vi "1WIRE_pulll_up_for_convert.vi"(8 "error in":errorcluster) -> (0 "error out":errorcluster)   [LabVIEW 2013]
doc: "This VI is created by Vincent Claes for FPDA-1 more information on http://pwo.fpga.be\n\nvincent.claes@xios.be\nclaesvincent@gmail.com\n\nhttp://www.linkedin.com/in/vincentclaes"
uses:
  <vilib>/eio/EIONode/EIONode.xnode
  <vilib>/eio/EIOMethodNode/EIOMethodNode.xnode
  <vilib>/rvi/eio/common/nirviEmuTemplateMethod_errors.vi
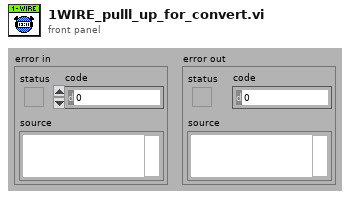
[diagram p1: front panel]
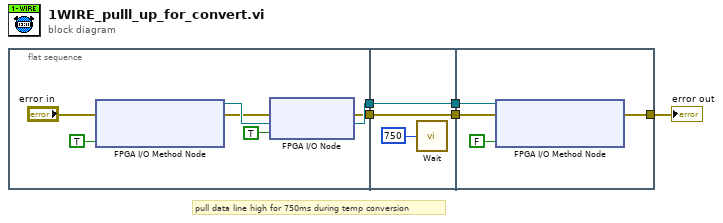
[diagram p0: block diagram]
diagram:
  # "pull data line high for 750ms during temp conversion"
  n1 = flat-sequence {
    tunnel: [w10] -> w5
    tunnel: [w7] -> w2
    tunnel: w5 -> [w14]
    tunnel: [w14] -> w4
    tunnel: [w13] -> w3
    tunnel: w2 -> [w13]
    tunnel: [w19] -> w1
    tunnel: w3 -> [w18]
    tunnel: w4 -> [w17]
    frame #0 {
      n2 = xnode "FPGA I/O Method Node"("error in"="error in", "Enable"=TRUE) -> ("error out"=w8:errorcluster, "FPGA I/O Out"=w11:refnum<k21>)  [unwired: 1 in]
      n3 = xnode "FPGA I/O Node"("error in"=w8, "I/O Item"=TRUE ("FX2_IO1_J1_0"), "FPGA I/O In"=w11) -> ("error out"=w7:errorcluster, "FPGA I/O Out"=w10:refnum<k21>)
    }
    frame #1 {
      n4 = call "Wait"("Count(mSec)"=u32 750 ("Count(uSec)")) -> ()  [unwired: 1 out]
    }
    frame #2 {
      n5 = xnode "FPGA I/O Method Node"("error in"=w18, "FPGA I/O In"=w17, "Enable"=FALSE) -> ("error out"=w19:errorcluster)  [unwired: 1 out]
    }
  }
  "error out" <- w1
